vi "Numato Command-Response.vi"(7 "VISA resource name":refnum<visa-resource-name>="COM4", 8 "error in (no error)":errorcluster, 11 "Command":string="relay writeall 0000") -> (0 "error out":errorcluster, 3 "Response":string)   [LabVIEW 2025, in "Interface Functions.lvlib"]
uses:
  <vilib>/Instr/_visa.llb/VISA Set IO Buffer Mask.ctl
  <vilib>/Instr/_visa.llb/VISA Configure Serial Port (Instr).vi
  Interface Functions.lvlib
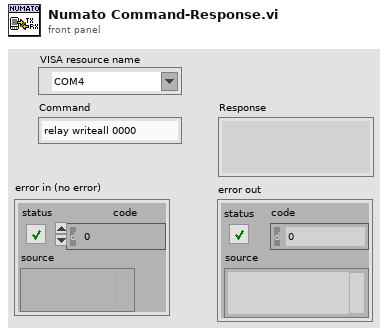
[diagram p1: front panel]
types:
  T1 = typedef "VISA Set IO Buffer Mask.ctl" = u16
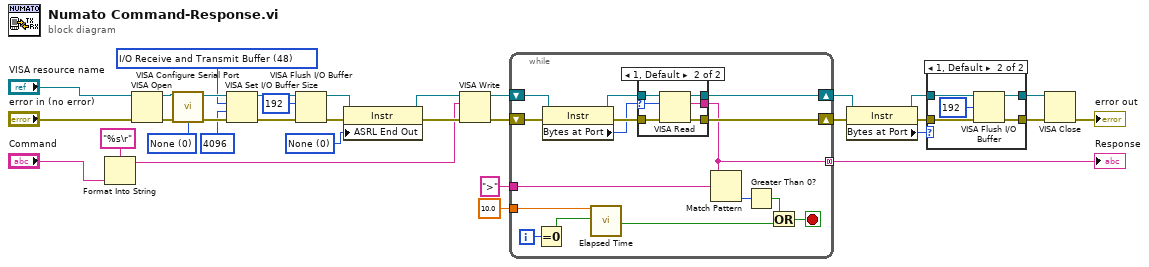
[diagram p0: block diagram]
diagram:
  w9 = u16 0 items=["None", "Last Bit", "TermChar", "Break"] ("Serial Settings:End Mode for Writes")
  w6 = T1 48 items=["I/O Receive Buffer"=16, "I/O Transmit Buffer"=32, "I/O Receive and Transmit Buffer"=48] ("Mask")
  w14 = u16 0 items=["None", "XON/XOFF", "RTS/CTS", "XON/XOFF & RTS/CTS", "DTR/DSR", "XON/XOFF & DTR/DSR"] ("flow control (0:none)")
  n1 = Format Into String(format string="%s\r", "Command") -> (resulting string=w7:string)  [unwired: 2 in, 1 out]
  n2 = VISA Open(error in (no error)="error in (no error)", VISA resource name="VISA resource name") -> (VISA resource name=w5:refnum<visa-resource-name>, error out=w4:errorcluster)  [unwired: 3 in]
  n3 = call-poly "VISA Configure Serial Port"("VISA resource name"=w5, "error in (no error)"=w4, "flow control (0:none)"=w14) -> ("VISA resource name out"=w16:refnum<visa-resource-name>, "error out"=w19:errorcluster)  [unwired: 11 in]
  n4 = VISA Set I/O Buffer Size(VISA resource name=w16, mask (16)=w6, size (4096)=u32 4096, error in (no error)=w19) -> (VISA resource name out=w17:refnum<visa-resource-name>, error out=w18:errorcluster)
  n5 = VISA Flush I/O Buffer(VISA resource name=w17, mask (16)=192, error in (no error)=w18) -> (VISA resource name out=w13:refnum<visa-resource-name>, error out=w12:errorcluster)
  n6 = property class="Instr"(reference=w13, error in=w12, "ASRL End Out"=w9) -> (reference out=w10:refnum<visa-resource-name>, error out=w11:errorcluster)
  n7 = VISA Write(VISA resource name=w10, write buffer=w7, error in (no error)=w11) -> (VISA resource name out=w32:refnum<visa-resource-name>, error out=w31:errorcluster)  [unwired: 1 out]
  n8 = while {
    shift-right: [w44] -> w27
    shift-left: w32 -> [w49]
    shift-right: [w45] -> w28
    shift-left: w31 -> [w48]
    tunnel: [w42] -> w23 mode=concatenating
    tunnel: ">" ("write buffer") -> [w43]
    tunnel: 10.0 ("Time Target (s)") -> [w39]
    i -> [w38]
    stop <- w40 stop-if-true
    n9 = Equal To 0?(x=w38) -> (x = 0?=w37:bool)
    n10 = property class="Instr"(reference=w49, error in=w48) -> (reference out=w47:refnum<visa-resource-name>, error out=w46:errorcluster, "Bytes at Port"=w35:u32)
    n11 = call "Elapsed Time"("Time Target (s)"=w39, "Reset"=w37) -> ("Time has Elapsed"=w36:bool)  [unwired: 10 in, 7 out]
    n12 = case shown="1, Default" w35 {
      selector: w35 -> [_ w52]
      tunnel: w47 -> [w51 w57]
      tunnel: w46 -> [w50 w56]
      tunnel: [w50 w55] -> w45
      tunnel: [w51 w54] -> w44
      tunnel: [_ w53] -> w42
      frame 0 {
      }
      frame 1, Default {
        n13 = VISA Read(VISA resource name=w57, byte count=w52, error in (no error)=w56) -> (VISA resource name out=w54:refnum<visa-resource-name>, read buffer=w53:string, error out=w55:errorcluster)  [unwired: 1 out]
      }
    }
    n14 = Match Pattern(string=w42, regular expression=w43) -> (offset past match=w41:i32)  [unwired: 1 in, 3 out]
    n15 = Greater Than 0?(x=w41) -> (x > 0?=w34:bool)
    n16 = Or(x=w34, y=w36) -> (x .or. y?=w40:bool)
  }
  "Response" <- w23
  n17 = property class="Instr"(reference=w27, error in=w28) -> (reference out=w25:refnum<visa-resource-name>, error out=w24:errorcluster, "Bytes at Port"=w26:u32)
  n18 = case shown="1, Default" w26 {
    tunnel: w25 -> [w59 w64]
    tunnel: w24 -> [w58 w63]
    tunnel: [w58 w61] -> w20
    tunnel: [w59 w60] -> w21
    frame 0 {
    }
    frame 1, Default {
      n19 = VISA Flush I/O Buffer(VISA resource name=w64, mask (16)=192, error in (no error)=w63) -> (VISA resource name out=w60:refnum<visa-resource-name>, error out=w61:errorcluster)
    }
  }
  n20 = VISA Close(VISA resource name=w21, error in (no error)=w20) -> (error out=→"error out":errorcluster)
